vi "Post-Processing VI Bin Files - LAMPS 8 Bit.vi"() -> ()   [LabVIEW 2016]
uses:
  <vilib>/Utility/config.llb/Read Key (I32).vi
  <vilib>/Utility/config.llb/Read Key (Double).vi
  <vilib>/Utility/config.llb/NI_LVConfig.lvlib
  Classes/Processing/Processing.lvclass
panel:
  in  "B Scan Select (Text Input)":i32=400
  out "Start Trim":dbl
  out "Stop Trim":dbl
  in  "A-Scan Change":i32=627
  out "BScan":u8[][](graph)
  out "Range":dbl=4.0
  out "Bits":dbl=16.0
  out "Points Per A Scan":i32=1600
  out "A-Scans Per BScan":i32=1000
  in  "Min / Max in dB (Contrast)":cluster{dbl, dbl}(slide)={-34.05144694533762, 14.823151125401928} scale=-40.0..60.0
  in  "Create 3D Data":bool=TRUE
  in  "Max":sgl=14.823152 format="%0.2f"
  in  "Min":sgl=-34.05145 format="%0.2f"
  out "Binary File Handle":refnum<file>
  in  "Create En Face Software Event":bool=TRUE
  out "En Face":sgl[][](graph)=[[-7.930091, -7.8040323, -7.973442, -8.000936, -7.8626037, -7.893125, -7.976362, -7.866958, -7.8874545, -8.053767, -7.895429, -8.001336, -8.058077, -7.9112062, -7.757364, -7.965038, -7.9575043, -8.167074, -8.054711, -8.167959, -7.8551683, -7.915979, -7.9114604, -7.864061, -8.055119, -7.9877367, -8.029805, -7.988413, -8.037094, -7.922483, -8.156847, -7.9672847, -7.8064103, -7.9114566, -7.773133, -7.9002914, -8.085471, -7.9221673, -7.957444, -7.958286, -7.698463, -8.002342, -7.989561, -7.952671, -7.984078, -7.836235, -8.0634165, -8.028308, -8.039231, -8.056543, -7.8877096, -7.9473996, -7.865986, -7.929803, -7.9396944, -7.8729186, -7.962053, -7.976538, -7.829268, -7.759593, -7.6770754, -7.917806, -7.978408, -7.7964263, -7.9014854, -7.8359327, -8.019228, -7.9651647, -7.961875, -8.0167675, -7.915086, -7.975068, -8.046566, -7.960596, -7.990237, -8.160412, -8.09407, -7.795923, -7.8977365, -7.917423, -8.06519, -7.941408, -8.036876, -7.946509, -8.009643, -7.7677317, -8.056414, -8.105821, -8.020063, -7.946077, -7.9010644, -8.056617, -8.010448, -8.0648775, -7.9236917, -7.8220835, -7.8197546, -7.8338175, -7.908895, -7.9036684, -7.9667068, -8.103706, -7.9954534, -7.9504957, -7.829475, -7.831149, -8.244316, -8.030985, -8.157568, -7.6754923, -7.9325967, -8.037667, -7.9114547, -7.946226, -7.8830395, -7.788606, -8.123245, -7.848808, -8.020647, -7.825039, -8.136002, -7.8881106, -7.840354, -7.8498588, -7.868983, -8.012706, -8.025735, -8.1118145, -7.816016, -7.8430986, -7.9750667, -8.042043, -7.820652, -7.8192554, -7.888372, -8.02898, -7.891756, -7.86369, -7.979582, -7.7987456, -8.169637, -7.8604546, -8.097469, -7.882909, -7.745224, -7.9409885, -8.008719, -7.874554, -7.934384, -7.889922, -7.9307194, -7.976539, -7.8116565, -8.037268, -7.8819757, -7.90127, -8.004612, -7.9514766, -7.6461873, -8.051855, -8.033362, -7.820009, -8.007025, -7.9113975, -7.972308, -8.075444, -7.9308887, -8.089264, -7.8016825, -7.919436, -7.94926, -7.7312274, -8.1581135, -7.806207, -7.956523, -7.9414477, -7.9876857, -7.9657526, -7.8116117, -7.8548036, -7.9839373, -7.9158034, -7.898539, -7.780124, -7.9533, -7.8764243, -7.739191, -7.80521, -8.063391, -7.9777446, -7.7854123, -7.9521074, -7.98957, -7.888753, -7.7991505, -7.9267855, -7.9612865, -7.819488, -7.865055, -8.14359, -7.7728977, -8.085733, -7.8384624, -7.743552, -7.886237, -7.9267993, -7.9535413, -7.8223243, -7.8396297, -7.870655, -8.026216, -7.7772164, -7.80645, -8.013777, -8.012371, -7.7353735, -7.935509, -7.860224, -7.9132657, -7.845752, -7.7870827, -7.958748, -8.160488, -7.869349, -7.78722, -7.955144, -7.8493533, -7.8096776, -7.986651, -7.945869, -7.935255, -8.144389, -7.9736667, -7.752922, -7.9255905, -7.974105, -7.799902, -7.6951523, -7.799085, -7.9162817, -8.017551, -7.9524965, -7.9512806, -8.165993, -7.7668185, -8.012505, -8.16206, -8.251981, -8.013035, -7.735666, -8.077859, -8.10991, -7.949526, -7.707088, -7.949591, -7.8823195, -7.816381, -8.034339, -7.868784, -7.89056, -7.8687153, -8.057175, -7.9518924, -7.9154468, -7.939955, -7.814576, -8.049959, -7.9097743, -7.863441, -7.846818, -7.96588, -7.789853, -8.094775, -7.7202816, -8.046873, -8.085813, -7.9780364, -7.9041257, -7.926487, -7.9343805, -8.040627, -7.830686, -8.070694, -7.8358226, -7.7780213, -7.8480616, -8.064976, -8.037013, -7.7728744, -8.012946, -7.9755006, -7.906261, -8.043798, -7.911961, -7.992775, -8.001271, -7.9195423, -8.082046, -8.020159, -7.9112606, -7.775108, -8.003549, -7.9803247, -7.8879714, -8.073655, -7.8865504, -7.783486, -7.8546762, -8.020269, -8.023449, -8.067884, -7.7598515, -7.90917, -8.069023, -7.7864647, -7.870191, -7.870761, -7.9444532, -7.993182, -7.917858, -8.03805, -7.93978, -7.7982545, -7.974645, -8.004379, -7.993704, -7.819672, -8.089255, -7.9242916, -7.907874, -7.9370337, -7.863256, -7.7989616, -7.80284, -8.006147, -7.823976, -7.995604, -8.050512, -7.964656, -8.11802, -7.9949827, -7.951066, -7.7912025, -7.927686, -8.008126, -7.891107, -8.10944, -8.134752, -7.8064127, -7.910995, -8.09849, -7.8788795, -8.016058, -7.8636923, -7.9307437, -7.974993, -7.991549, -7.974662, -7.93784, -7.7311897, -8.182317, -7.7587895, -8.095182, -7.874478, -7.813459, -7.879261, -7.829288, -8.035134, -7.861396, -7.986878, -7.782207, -7.79948, -7.9310637, -7.852276, -7.9916263, -7.9213424, -8.203527, -7.921085, -8.025147, -7.8967156, -7.8208995, -7.9961405, -8.083003, -7.98257, -7.9804964, -7.8674, -8.060883, -7.9558725, -7.945471, -8.142715, -8.087639, -8.218578, -8.243896, -7.959839, -7.9356184, -7.7503934, -8.0898695, -7.868658, -7.692663, -7.887905, -7.8621182, -7.9225054, -7.836562, -8.054047, -7.982782, -7.744281, -7.963519, -8.0447, -7.849429, -7.838456, -8.119481, -7.7900977, -7.9761267, -7.8695583, -7.76462, -7.970638, -7.9605556, -7.964503, -7.9509263, -7.86703, -8.055239, -7.884155, -7.844713, -7.856759, -7.9913874, -8.0371475, -7.938692, -8.049144, -8.021844, -7.7414804, -7.920646, -8.197608, -7.880194, -7.9744005, -8.035382, -8.069501, -8.181021, -8.0188465, -8.004074, -8.031586, -8.0189085, -8.058473, -7.9364552, -7.719303, -7.905371, -7.790757, -8.214631, -7.9018154, -7.987326, -7.9526286, -7.8612223, -7.9100804, -8.08193, -7.9836636, -8.027385, -8.095275, -7.9418774, -7.9966297, -7.9296713, -8.01897, -7.9224367, -7.8740377, -7.8067255, -8.113648, -7.965984, -7.919392, -7.9538283, -7.9669385, -7.9489245, -7.9807835, -8.049196, -8.2190485, -7.967722, -8.009465, -7.814837, -7.9246864, -7.923164, -7.990351, -7.917373, -8.095252, -8.055175, -8.003493, -7.828865, -7.96325, -7.9371457, -7.87614, -7.833712, -8.081883, -7.9843564, -7.8006735, -7.917411, -7.8912277, -7.9116125, -8.126464, -7.9357214, -7.9421554, -7.757199, -7.938931, -7.852307, -8.009288, -7.8433046, -7.8127127, -7.774231, -7.958359, -7.8807616, -8.237229, -8.159578, -7.96494, -8.140689, -7.666607, -7.9215274, -7.7746763, -7.9678416, -8.0088625, -7.897964, -7.9378257, -8.099062, -8.039701, -7.9717793, -8.185365, -8.0567465, -7.9489536, -7.8975363, -8.023378, -7.8149986, -7.7747483, -8.115946, -8.063846, -7.8867245, -7.9420667, -7.8944864, -8.023156, -7.8669634, -7.876997, -7.841495, -7.9707136, -7.9111295, -7.863631, -8.016624, -7.956105, -7.858278, -8.059558, -8.096037, -7.892564, -7.9129233, -7.79077, -7.9832497, -7.985417, -7.7849727, -8.001589, -7.7398777, -7.7428336, -7.906874, -8.126725, -8.015352, -8.038417, -7.965966, -7.911179, -7.9052196, -7.9147563, -7.75231, -8.021024, -7.8436966, -8.057442, -7.9307613, -7.822249, -8.146226, -8.007187, -7.6794977, -7.83178, -7.8921013, -8.013386, -8.003119, -7.9583955, -7.938617, -8.110327, -8.210196, -7.9229064, -7.970181, -7.8199425, -8.0372505, -7.8034477, -7.8715796, -8.105112, -7.8673153, -7.9806876, -7.944533, -7.8558373, -8.031324, -8.0394125, -7.9362345, -7.8742948, -8.004431, -7.9117155, -7.92383, -8.22453, -7.9384084, -8.046981, -7.948592, -7.9943843, -8.039814, -7.867514, -7.8567586, -7.7503667, -8.132967, -7.8055544, -8.099513, -8.015846, -7.80609, -8.167438, -7.801515, -7.9792643, -7.9695144, -7.709452, -7.8683558, -7.7977037, -7.904273, -7.790883, -8.073817, -8.044217, -7.6886067, -7.854426, -7.841001, -7.8545475, -8.139268, -7.948963, -7.89186, -7.8355184, -7.917378, -7.9529567, -7.8986993, -7.7398877, -7.946703, -7.9786987, -8.031789, -7.9741163, -7.870274, -7.9702334, -8.02977, -7.8809557, -7.8097644, -7.9288607, -8.126841, -7.8123865, -7.8626604, -7.8187237, -7.8525906, -7.9653254, -7.9950914, -7.9080153, -8.03097, -7.805545, -7.777243, -7.77037, -8.001218, -8.017348, -8.007549, -7.8903728, -7.851192, -7.73721, -7.894369, -7.9804764, -7.972263, -8.017426, -7.9188137, -7.699553, -7.985173, -8.14926, -7.9460635, -7.9795494, -8.0467, -7.855538, -7.912811, -7.9511986, -7.9749317, -7.9023323, -7.9952846, -7.9592586, -8.030751, -7.920987, -7.924575, -7.641929, -7.819344, -7.847093, -7.996105, -7.60953, -7.8648734, -8.019921, -7.804081, -7.8468595, -7.806482, -7.854887, -7.9134655, -7.771183, -7.8451014, -8.077572, -8.037743, -7.8422785, -8.027252, -7.953315, -7.8755074, -7.9896126, -7.8166866, -8.076665, -7.956374, -8.030051, -7.9240355, -7.884757, -7.8483443, -7.8289475, -8.139085, -7.770633, -7.9318833, -8.016564, -7.8698854, -7.7932873, -7.8172855, -7.8905444, -7.986914, -7.9401693, -7.9614263, -7.9716263, -7.9189005, -8.085335, -7.7258472, -8.012342, -7.7290063, -7.962374, -7.736857, -7.908464, -7.95836, -7.727169, -7.9340315, -8.031877, -7.887279, -7.8412385, -8.041202, -7.8045454, -7.8905506, -7.7506995, -7.9316373, -7.9499393, -7.851978, -7.9120736, -7.9021235, -7.8550596, -7.8048263, -7.946267, -8.050364, -7.9034224, -7.9725904, -7.869547, -7.885991, -7.968221, -7.78149, -7.824945, -7.8112597, -7.997913, -8.123039, -7.8428135, -8.064973, -7.86549, -7.898531, -7.871154, -7.8630815, -8.026972, -8.056086, -8.107686, -7.9592414, -7.802565, -7.8990717, -7.8917937, -7.9946303, -7.935857, -7.7870903, -7.925476, -8.08807, -7.9506598, -7.903563, -7.7953897, -7.938492, -7.7871675, -7.921679, -7.8528447, -8.03581, -7.8427415, -7.889442, -7.972731, -8.008952, -7.9870386, -7.81934, -8.098788, -7.990713, -7.902563, -8.00334, -8.157312, -7.8009663, -7.755303, -8.165585, -8.05285, -7.908865, -7.8209777, -7.978314, -7.8780475, -7.93847, -7.8299446, -7.8623195, -7.93139, -7.7586055, -7.9444237, -7.8643084, -7.877962, -8.007582, -7.7742763, -7.890612, -8.051581, -7.892482, -7.8677154, -7.927973, -7.8819814, -7.9347353, -7.999919, -8.090686, -7.8633533, -7.88977, -8.057978, -8.034815, -7.7877083, -7.817199, -7.9679923, -8.017427, -7.9522886, -7.943636, -7.9850945, -7.99855, -7.863006, -7.88045, -8.068299, -7.925362, -8.142173, -7.8893266, -7.957223, -7.7491736, -7.852534, -8.071495, -7.865574, -7.799149, -7.8367667, -7.996641, -8.050482, -8.003815, -7.783416, -8.051039, -7.9302397, -8.008375, -7.833727, -7.8489013, -7.9530954, -7.9982214, -7.953154, -7.9360614, -8.100909, -7.979594, -7.670946, -8.022225, -7.8406134, -8.0095, -8.040179, -7.865175, -7.9610953, -8.07941, -7.9528823, -7.8656754, -7.979678, -7.802908, -7.972213, -7.9385486, -8.097144, -7.7224145, -7.8400908, -7.9734745, -8.105193, -7.8446107, -7.968687, -7.7581, -8.128169, -8.130323, -7.7925196, -8.015969, -7.678966, -7.872306, -7.836657, -7.9079814, -7.84879, -8.133352, -7.889341, -8.066047, -7.982547, -7.951533, -7.902655, -8.105811, -7.97907, -7.9479356, -7.960124, -7.8474517, -8.111724, -7.9724307, -7.975754, -7.985938, -7.9817557, -7.78798, -8.040827, -7.760837, -7.8727965, -7.984424, -8.078643, -7.885198, -7.9081254, -7.7833333, -7.908534, -7.6961055, -7.913281, -7.7185884, -8.042309, -8.115078, -8.14631, -7.806838, -7.7963495, -8.055587, -7.97538, -7.698462, -7.775273, -8.045425, -8.037591, -8.0973015, -7.7711625, -7.988266, -7.9091988, -7.8253546, -7.925254, -7.9461355, -7.766041, -7.8593016, -7.9350066, -8.008051, -7.861942, -7.8998094, -8.016808, -8.124489, -7.9874635, -8.083402, -8.1051035, -7.993055, -7.880184, -7.91285, -7.9538074, -7.9280205, -8.043174, -8.137445, -8.110672, -7.897486, -7.9666576, -7.978455, -7.9780507, -8.032585, -8.116778, -7.971109, -7.824977, -7.766515, -7.981128, -7.930899, -8.109892, -7.9214025, -7.8610687, -7.839897, -8.006488, -7.792739, -7.9065375, -8.032204, -7.81708, -7.790314, -8.064906, -8.093157, -7.839383, -8.11415, -7.9893, -8.070883, -8.176108, -7.7919936, -8.105036, -8.017701, -8.068903, -8.093538, -7.8479977, -7.9812527, -7.871276, -7.8107314, -7.958203, -7.8588, -7.829434]]
  out "error out":errorcluster
  in  "En Face Upper Depth":i32=60
  in  "En Face Lower Depth":i32=300
  in  "B-Scan Select":i32(slide) scale=0.0..1.0
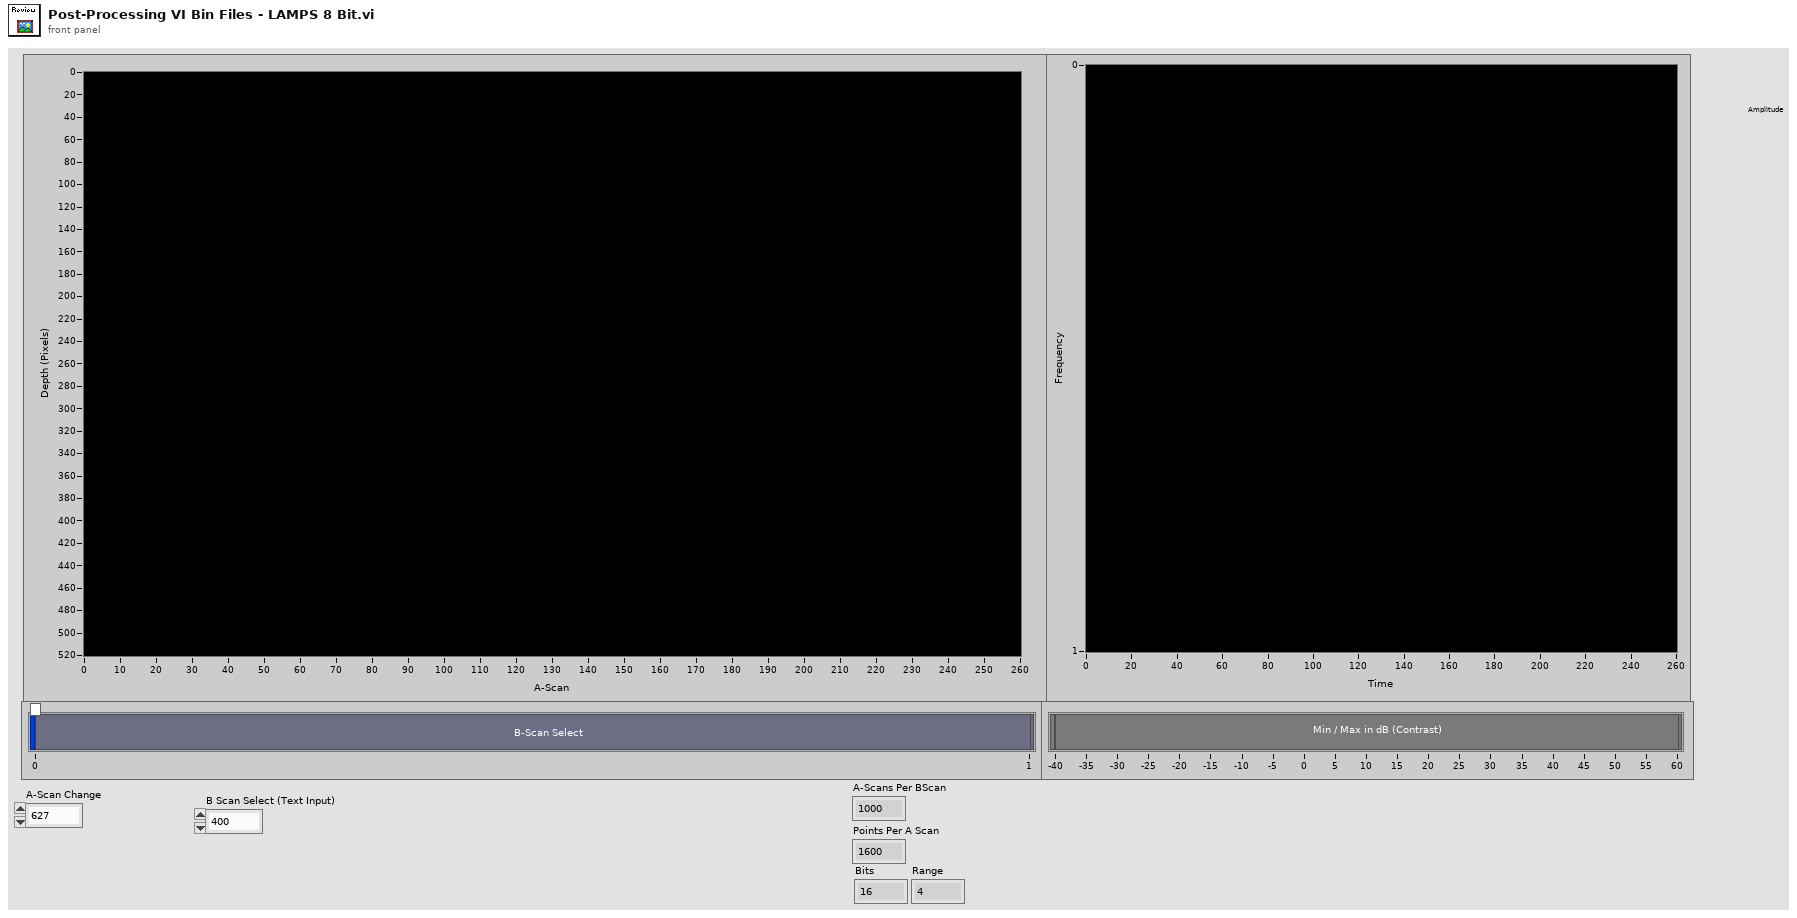
[diagram p1: front panel]
types:
  T1 = enum32{"Invalid", "Standard", "Closed", "Hidden", "Minimized", "Maximized"}
  T2 = typedef "NI_LVConfig.lvlib/Config Data RefNum.ctl" = refnum<k1>
  T3 = typedef "imagedata.ctl" = cluster{"image type":i32, "image depth":i32, "image":u8[], "mask":u8[], "colors":u32[], "Rectangle":cluster{"left":i16, "top":i16, "right":i16, "bottom":i16}}
  T4 = typedef "LVCursorListTypeDef.ctl" = cluster{"Name":string, "Color":u32, "Style":u8, "Point Style":u8, "Name Visible":bool, "Allow Drag":bool, "Cursor Mode":u32, "Plot":i32, "Index":i32, "Position":cluster{"X":dbl, "Y":dbl}, "X Scale":u32, "Y Scale":u32, "Watch Plots":i32[], "Watch All Plots":bool, "Plot Area":i32, "Label Offset":cluster{"X":dbl, "Y":dbl}}[]
  T5 = cluster{"Name":string, "Color":u32, "Style":u8, "Point Style":u8, "Name Visible":bool, "Allow Drag":bool, "Cursor Mode":u32, "Plot":i32, "Index":i32, "Position":cluster{"X":dbl, "Y":dbl}, "X Scale":u32, "Y Scale":u32, "Watch Plots":i32[], "Watch All Plots":bool, "Plot Area":i32, "Label Offset":cluster{"X":dbl, "Y":dbl}}
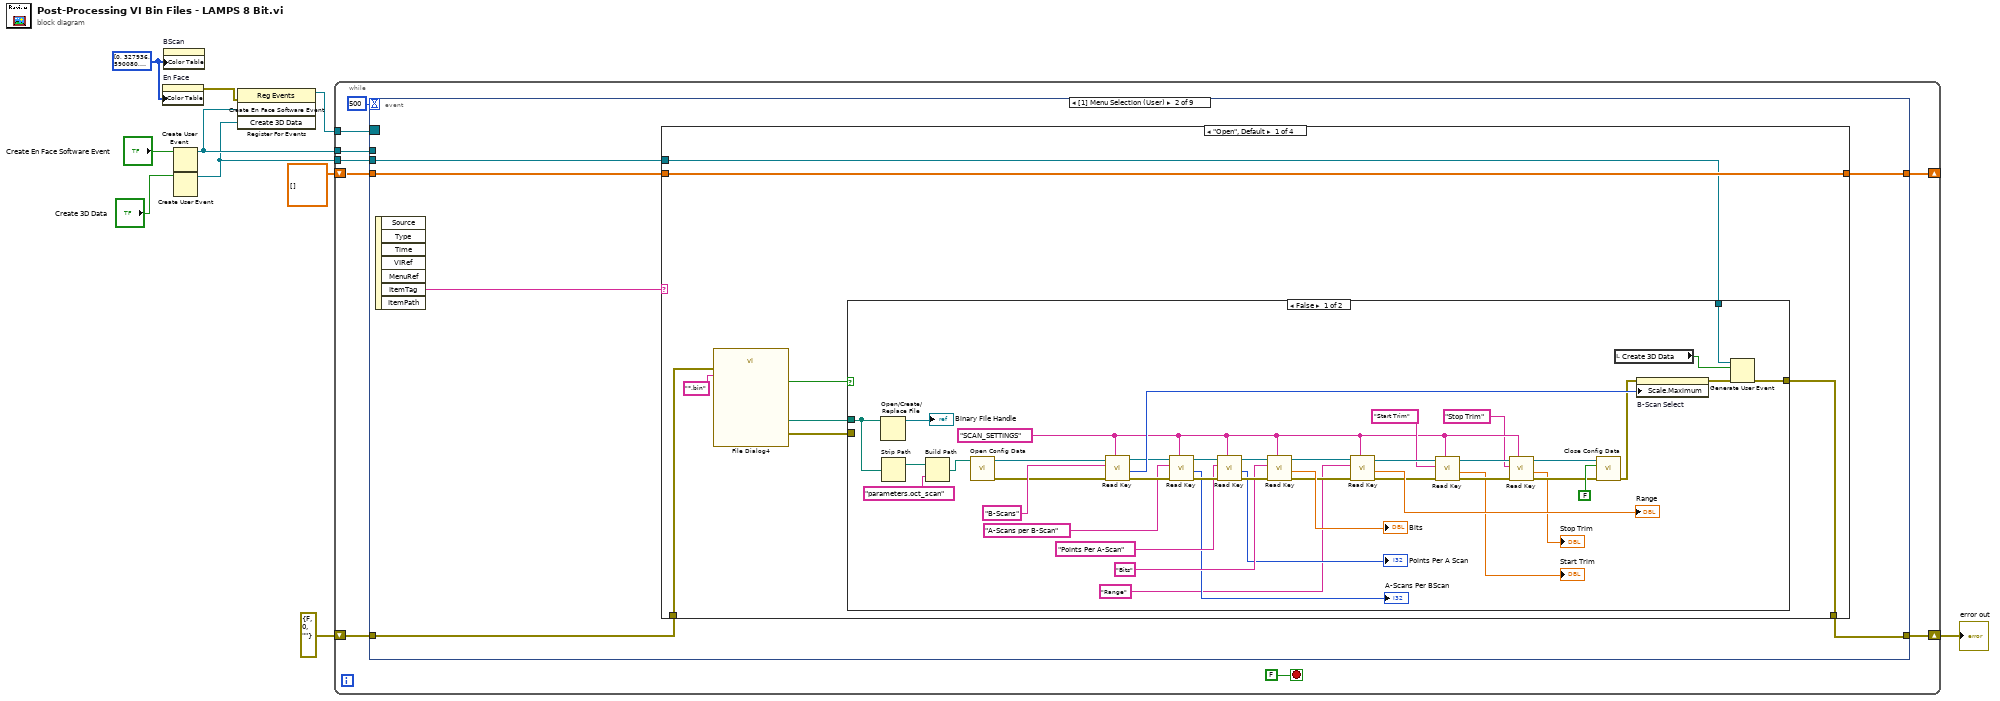
[diagram p0: block diagram]
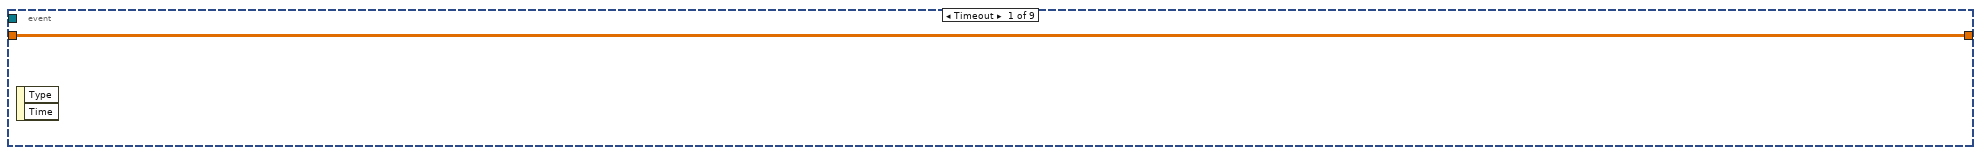
[diagram p2: hidden frame]
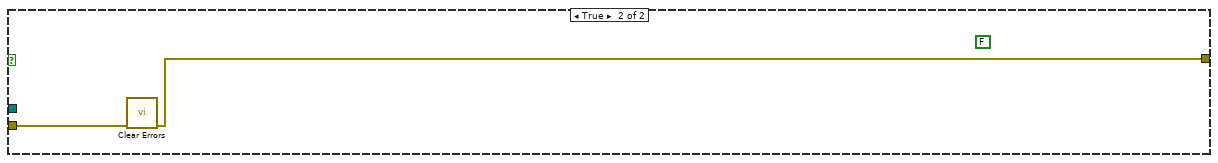
[diagram p3: hidden frame]
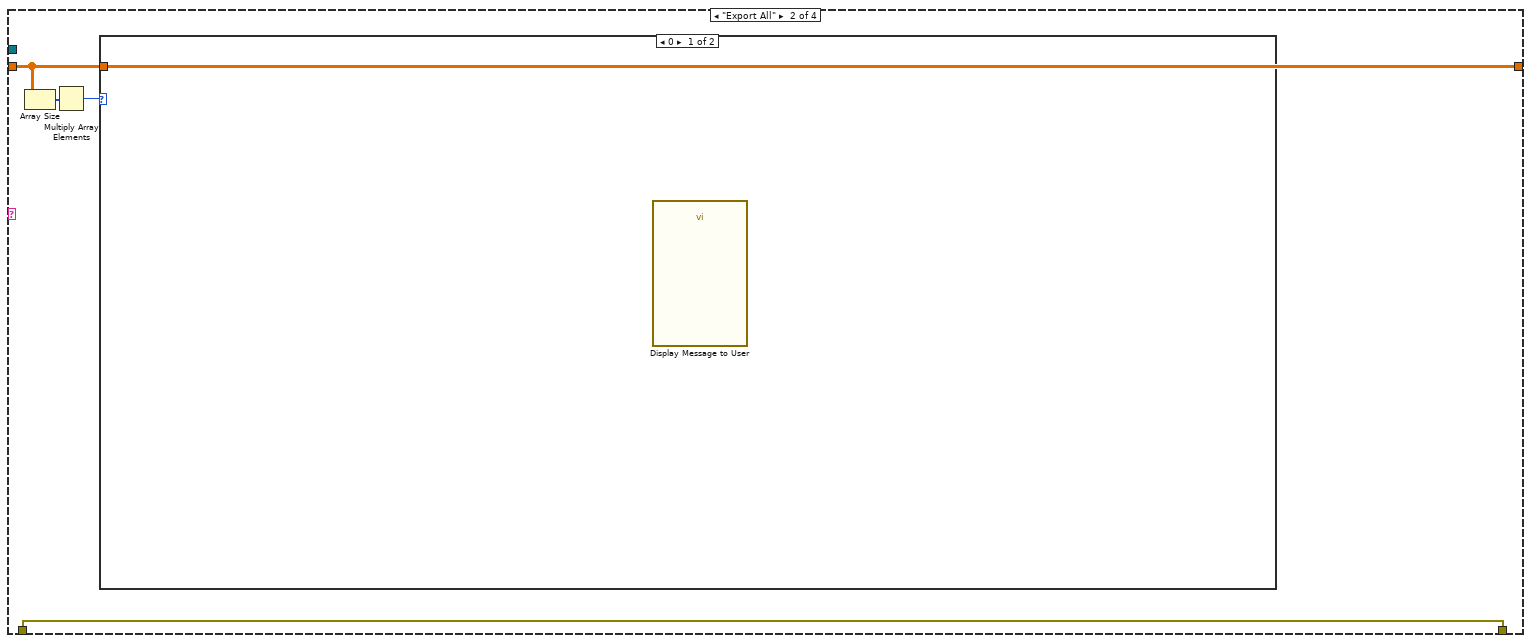
[diagram p4: hidden frame]
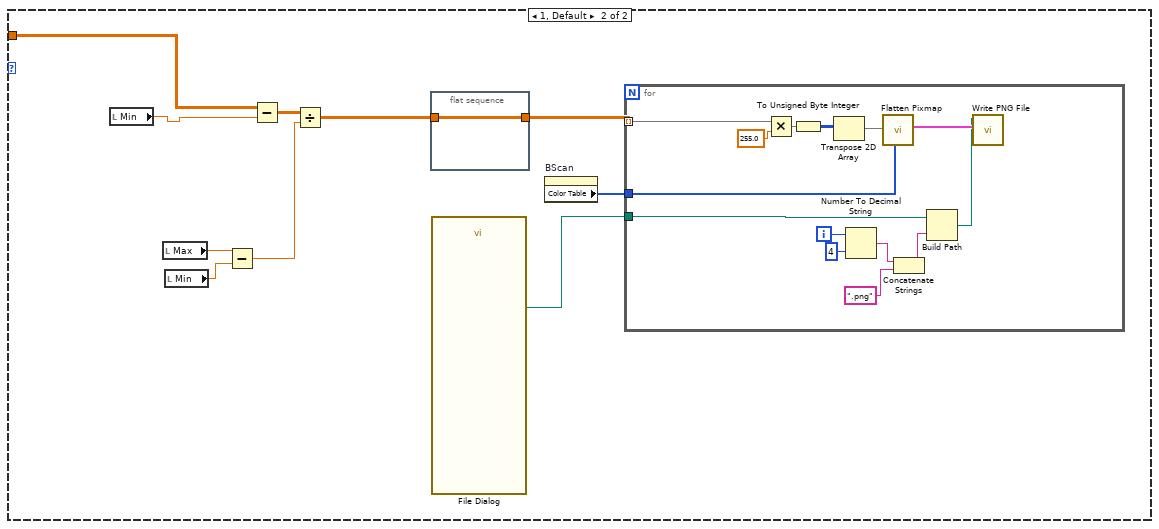
[diagram p5: hidden frame]
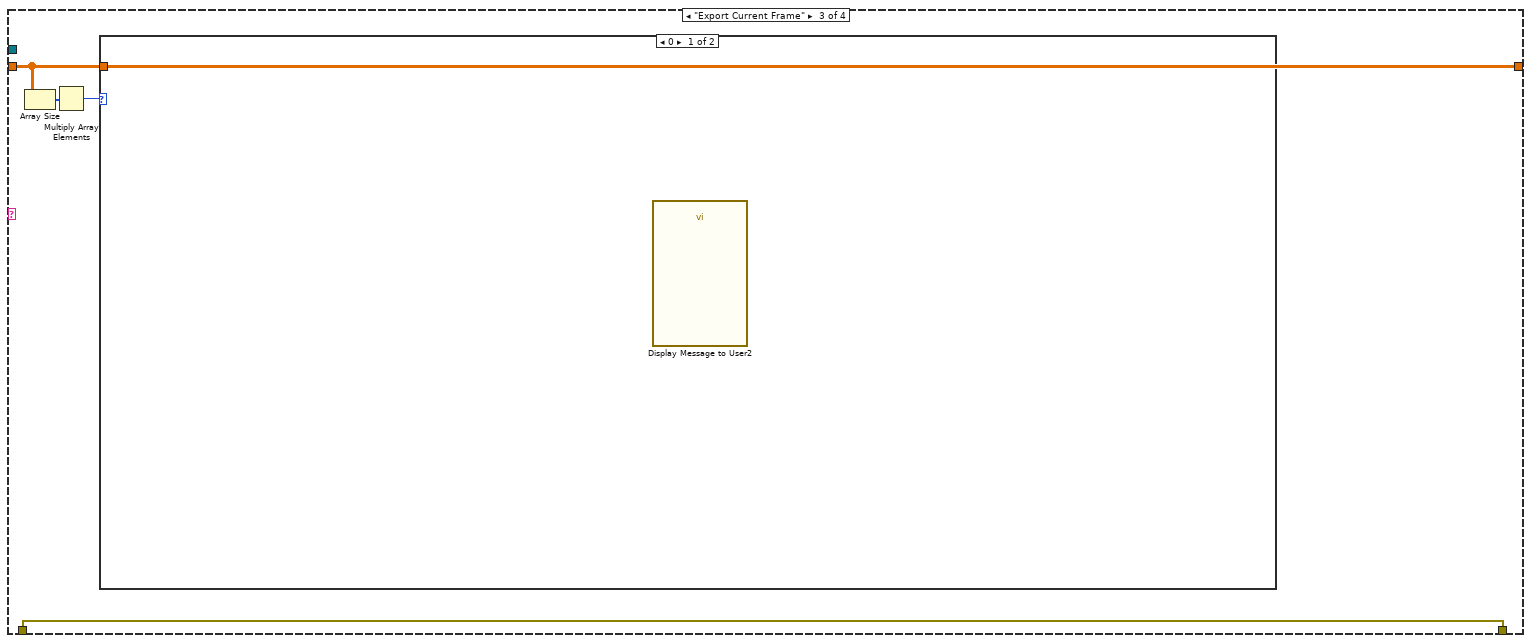
[diagram p6: hidden frame]
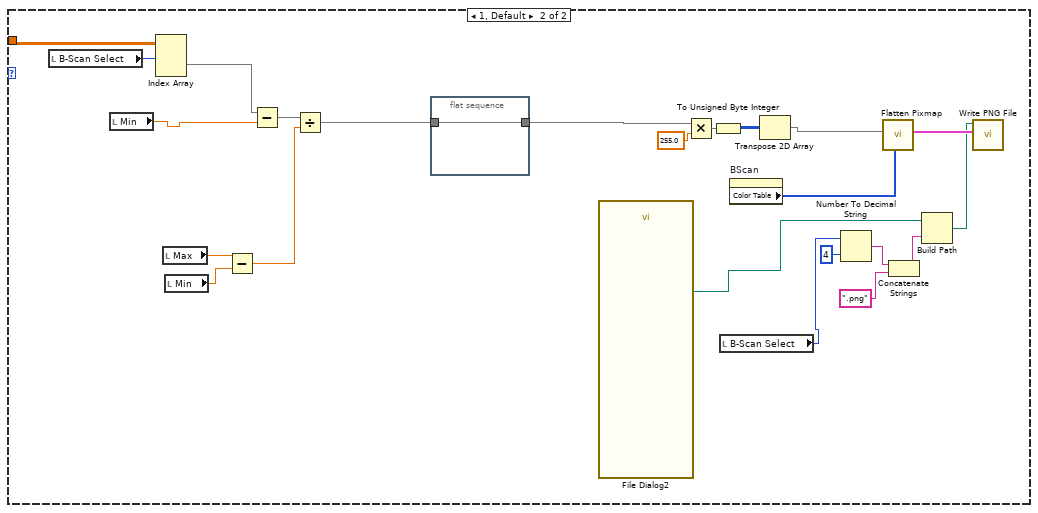
[diagram p7: hidden frame]
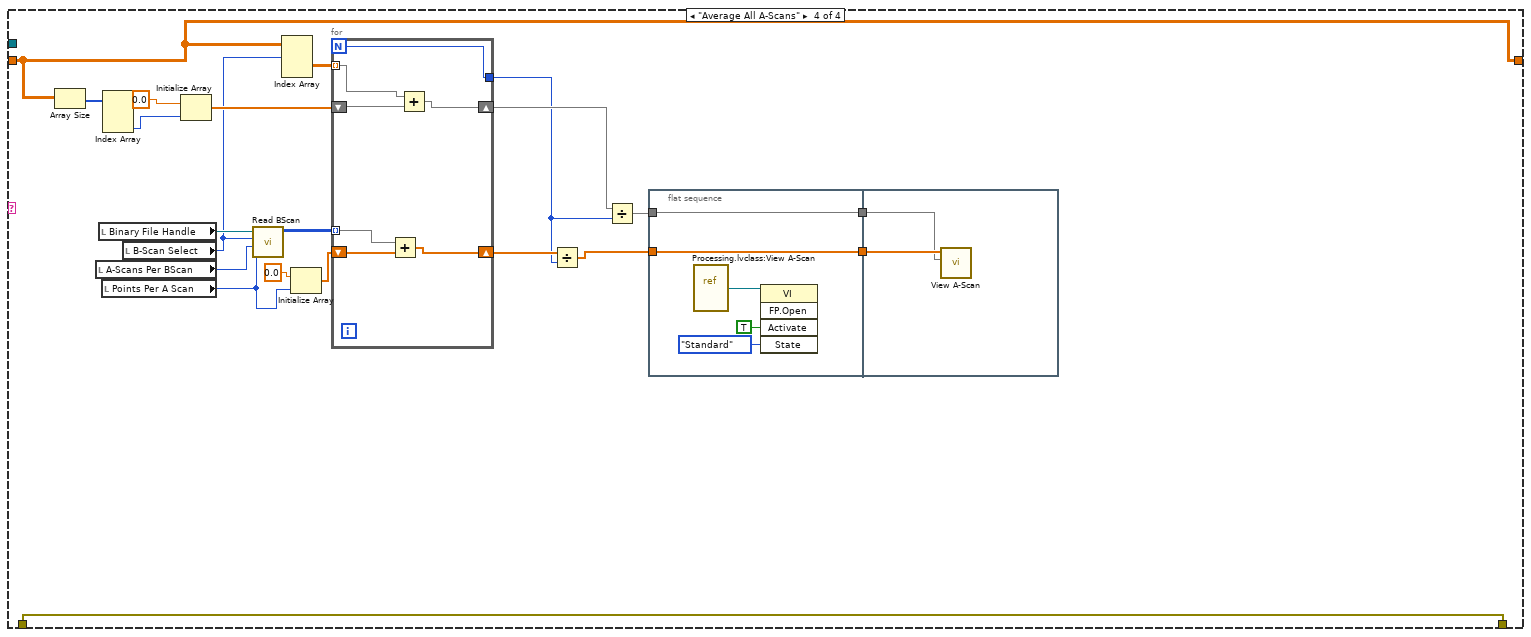
[diagram p8: hidden frame]
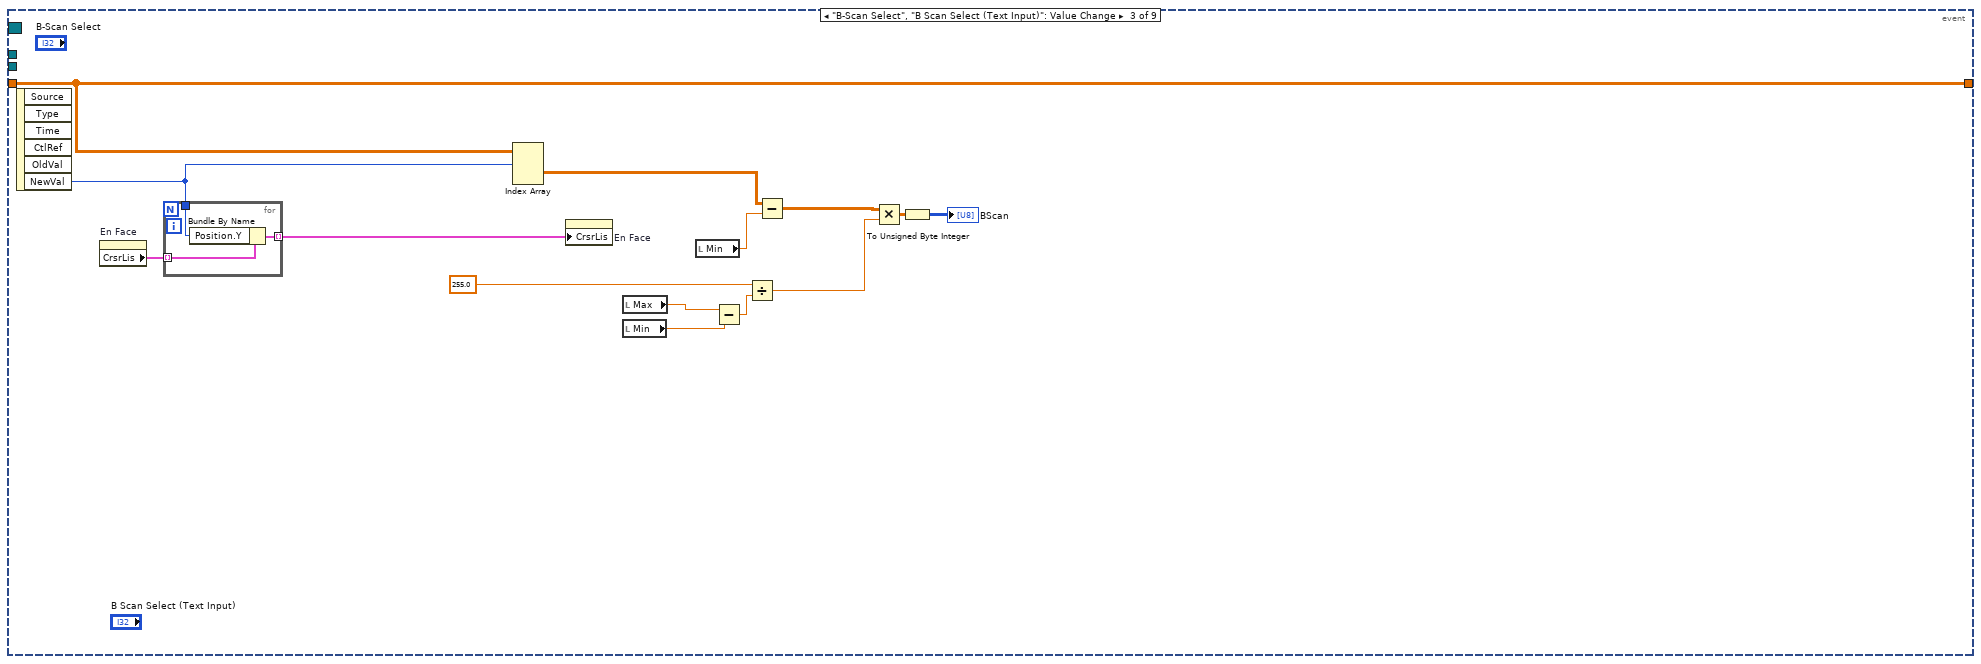
[diagram p9: hidden frame]
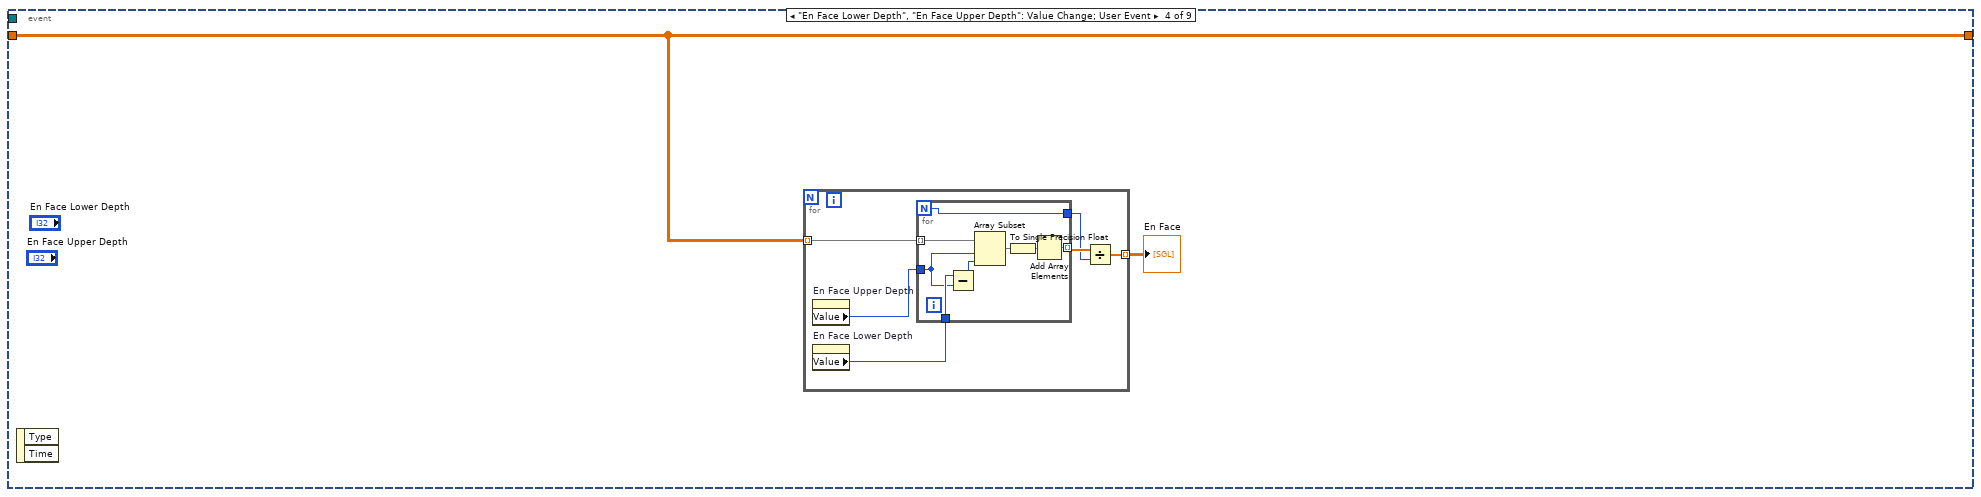
[diagram p10: hidden frame]
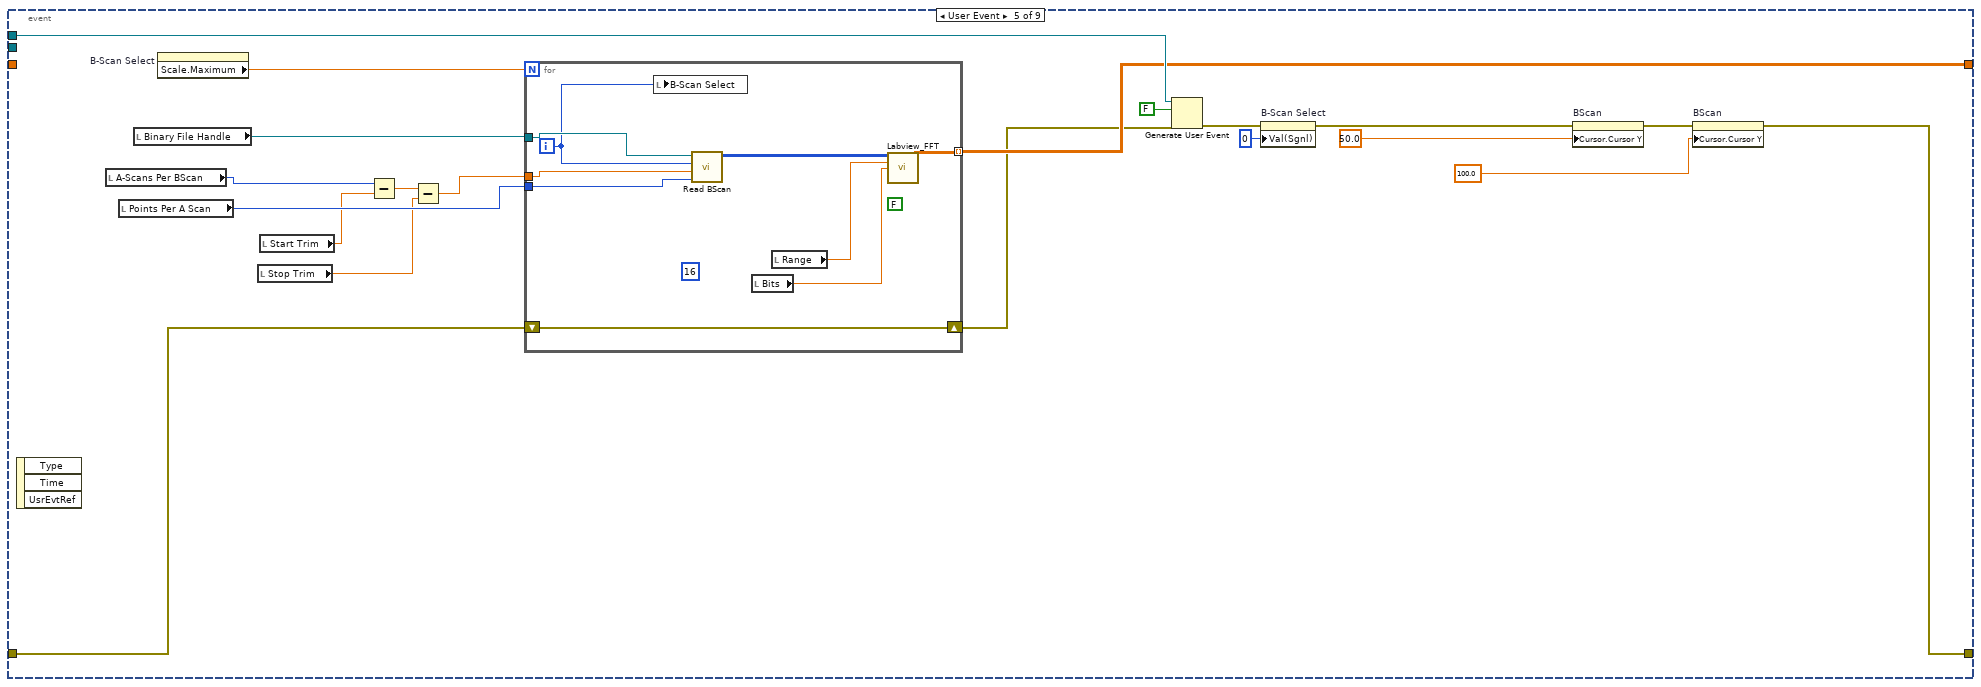
[diagram p11: hidden frame]
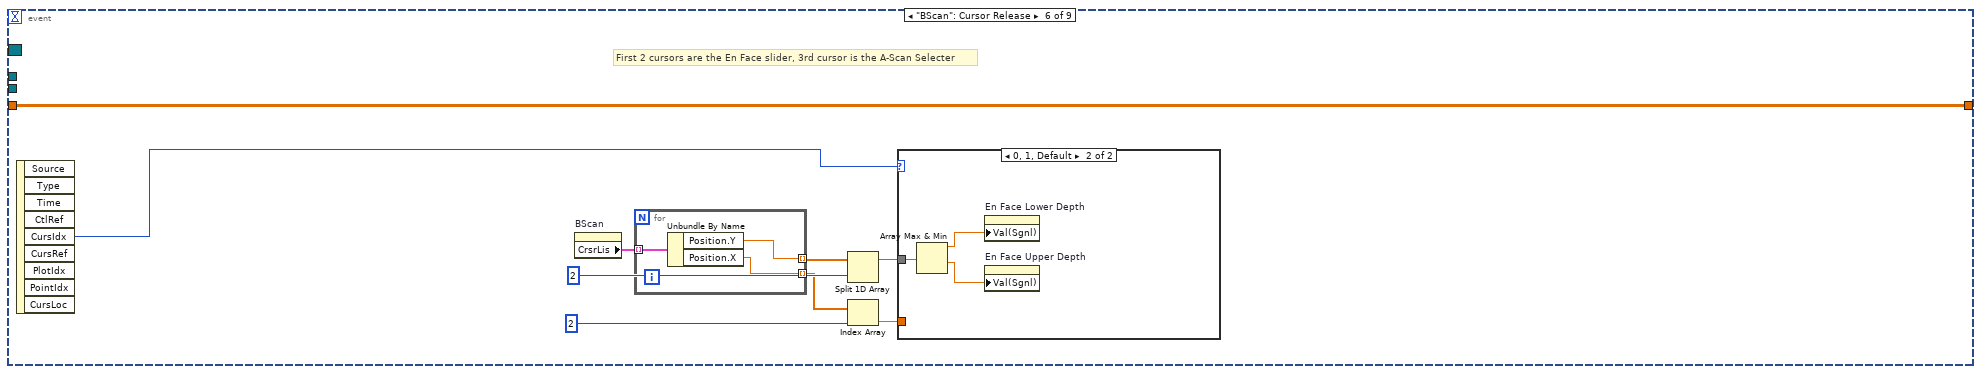
[diagram p12: hidden frame]
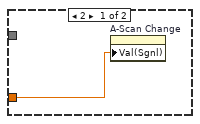
[diagram p13: hidden frame]
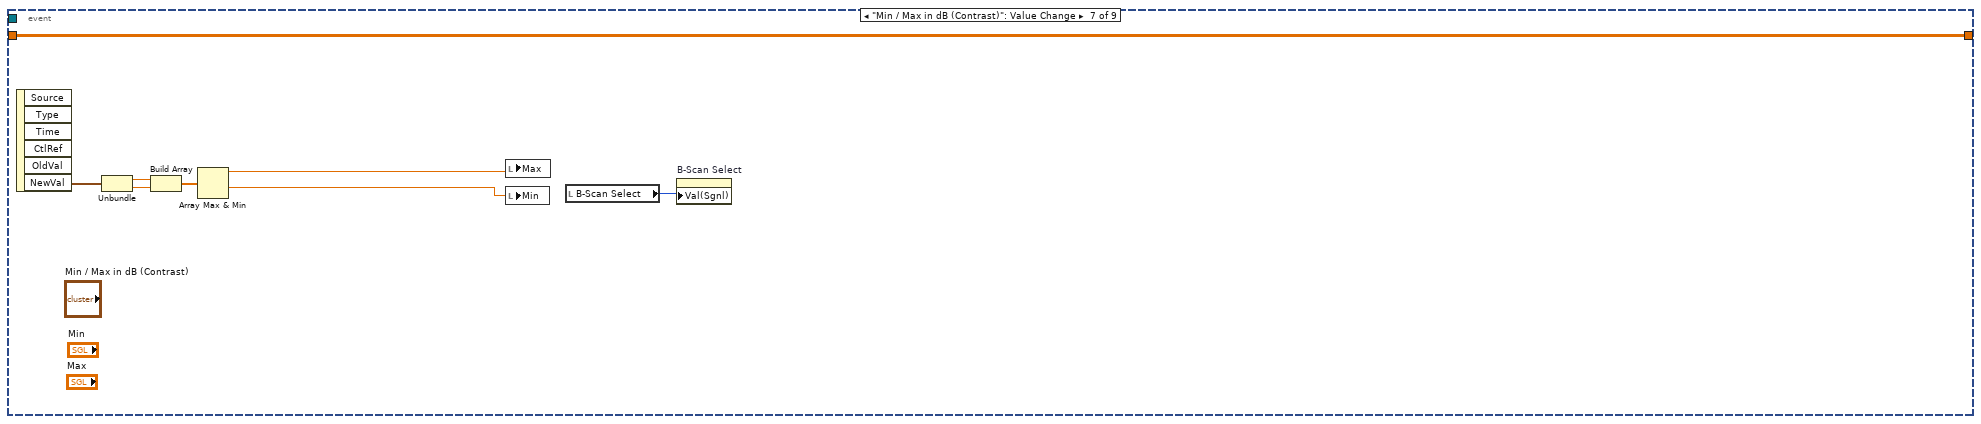
[diagram p14: hidden frame]
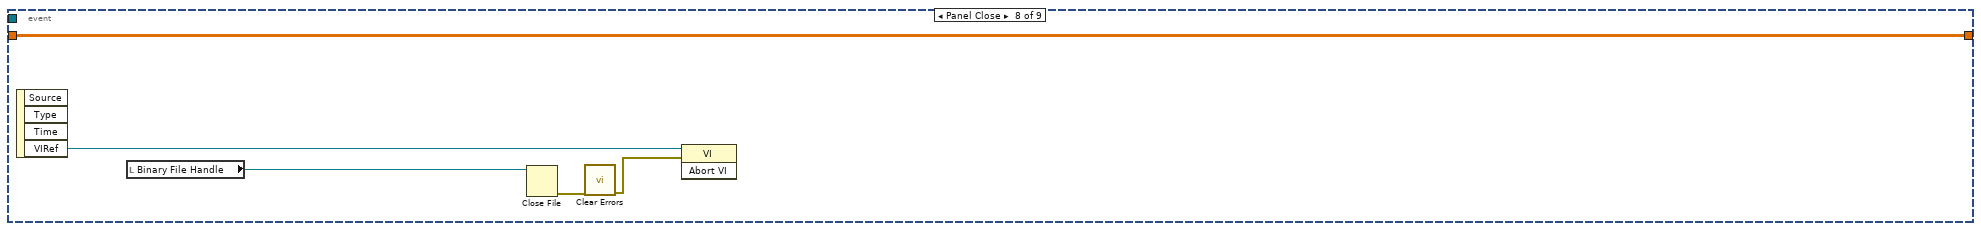
[diagram p15: hidden frame]
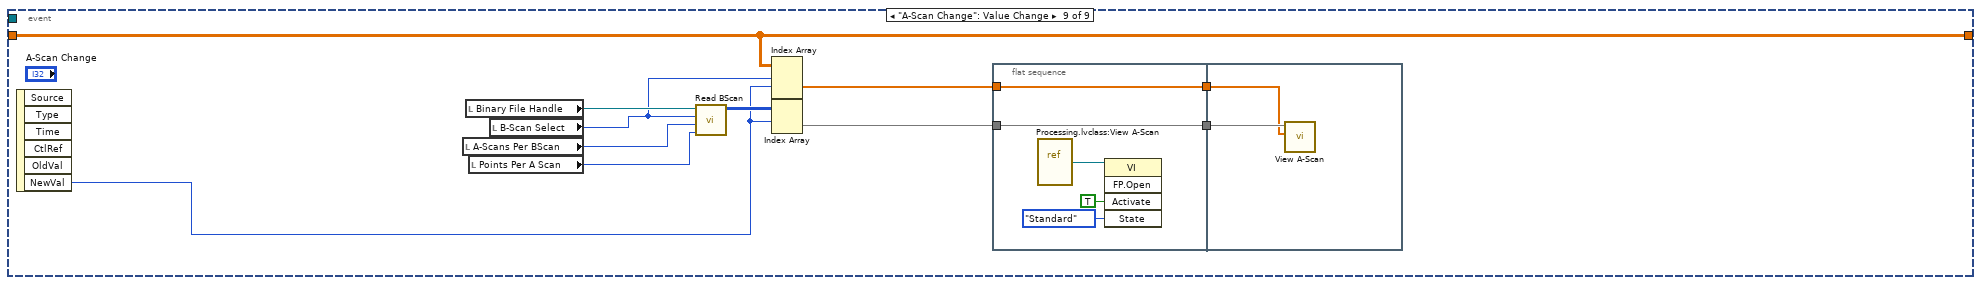
[diagram p16: hidden frame]
diagram:
  w3 = u32[] [0, 327936, 590080, 852224, 983296, 1114624, 1180160, 1311232, 1442304, 1573632, 1704704, 1770240, 1901312, 1966848, 2098176, 2163712, 2294784, 2491392, 2557184, 2688256, 2753792, 2884864, 2950656, 3081728, 3147264, 3344129, 3475457, 3540993, 3672321, 3738113, 3869185, 3934977, 4066305, 4197633, 4328961, 4394497, 4460289, 4591617, 4657409, 4788481, 4854273, 4985601, 5116929, 5248257, 5314049, 5379841, 5511169, 5576961, 5708033, 5773825, 5905153, 6036482, 6167810, 6233346, 6299138, 6430466, 6496258, 6562050, 6693634, 6759426, 6890754, 7022082, 7087874, 7153666, 7284994, 7350786, 7482114, 7547906, 7613698, 7745026, 7876354, 8007682, 8073474, 8139522, 8205314, 8336642, 8467970, 8533763, 8599555, 8665347, 8731139, 8862467, 8993795, 9059587, 9125380, 9191428, 9257220, 9388548, 9454340, 9520132, 9585924, 9717253, 9848837, 9914629, 9980165, 10045957, 10177541, 10243334, 10309126, 10375174, 10440966, 10572294, 10703623, 10769416, 10835208, 10901256, 10967049, 11033097, 11033609, 11099401, 11165450, 11231242, 11231754, 11297547, 11363339, 11429131, 11495180, 11495692, 11561740, 11693069, 11758861, 11759373, 11825165, 11891214, 11957006, 12022799, 12023311, 12089103, 12220944, 12286736, 12286736, 12352529, 12418577, 12484370, 12550162, 12615954, 12681747, 12747796, 12813588, 12813845, 12879894, 12945686, 13077015, 13142808, 13143064, 13208856, 13274905, 13340697, 13340953, 13472282, 13538075, 13604379, 13670172, 13735964, 13801757, 13867550, 13933343, 13999392, 13999648, 14065441, 14131234, 14197027, 14197541, 14263334, 14329383, 14395176, 14460969, 14592553, 14658346, 14724139, 14789932, 14790189, 14856238, 14922287, 14988080, 15053873, 15054130, 15119923, 15185972, 15251765, 15317559, 15383353, 15449146, 15449660, 15515454, 15515968, 15516226, 15582021, 15582278, 15582536, 15648587, 15648844, 15714639, 15714897, 15715155, 15780949, 15781463, 15847256, 15847770, 15848028, 15913823, 15914081, 15979875, 15980133, 15980391, 16046441, 16046444, 16046703, 16046705, 16112500, 16113015, 16113274, 16113277, 16179072, 16179330, 16179588, 16245384, 16245387, 16245389, 16245648, 16311443, 16376982, 16377241, 16377499, 16443294, 16443553, 16443555, 16443815, 16509866, 16510124, 16510127, 16575923, 16575924, 16576182, 16576441, 16576443, 16576702, 16576705, 16576963, 16577222, 16577224, 16577482, 16577485, 16577743, 16577745, 16578004, 16578262, 16578264, 16578523, 16578782, 16579040, 16579299, 16579301, 16579303, 16579562, 16579821] ("Color Table")
  n1 = property on="En Face" class="IntGraph (strict)"("Color Table"=w3) -> (error out=w2:errorcluster)  [unwired: 2 in, 1 out]
  n2 = property on="BScan" class="IntGraph (strict)"("Color Table"=w3) -> ()  [unwired: 2 in, 2 out]
  n3 = Create User Event(user event datatype="Create En Face Software Event") -> (user event=w9:refnum<user-event>)  [unwired: 1 in, 1 out]
  n4 = Create User Event(user event datatype="Create 3D Data") -> (user event=w8:refnum<user-event>)  [unwired: 1 in, 1 out]
  n5 = register-events(error in=w2, w9, w8) -> (reference out=w10:refnum<event-registration>)  [unwired: 1 in, 1 out]
  n6 = while {
    tunnel: w10 -> [w17]
    tunnel: w9 -> [w16]
    tunnel: w8 -> [w15]
    shift-right: [w13] -> w4
    shift-left: errorcluster {"status"=FALSE, "code"=0, "source"=""} ("error constant") -> [w14]
    shift-right: [w11] -> _
    shift-left: sgl[][][] [] ("Int B-Scan Channel A") -> [w12]
    stop <- FALSE stop-if-true
    n7 = event shown="[1] Menu Selection (User)" {
      selector: w17 -> [_ _ _ _ _ _ _ _ _]
      dyn-events: _ -> [_ _ _ _ _ _ _ _ _]
      timeout: 500 -> [_ _ _ _ _ _ _ _ _]
      tunnel: w15 -> [_ w23 _ _ _ _ _ _ _]
      tunnel: w16 -> [_ _ _ _ w220 _ _ _ _]
      tunnel: w14 -> [_ w22 _ _ w219 _ _ _ _]
      tunnel: [_ w21 _ _ w212 _ _ _ _] -> w13
      tunnel: w12 -> [w20 w25 w172 w188 _ w241 w249 w260 w268]
      tunnel: [w20 w24 w172 w188 w216 w241 w249 w260 w268] -> w11
      event Timeout {
        n8 = event-data() -> ()  [unwired: 1 in, 2 out]
      }
      event Menu Selection (User) {
        n9 = event-data() -> ("ItemTag"=w26:string)  [unwired: 1 in, 6 out]
        n10 = case shown="\"Open\", Default" w26 {
          tunnel: w25 -> [w34 w81 w110 w149]
          tunnel: [w34 w81 w110 w149] -> w24
          tunnel: w23 -> [w28 _ _ _]
          tunnel: w22 -> [w31 w82 w111 w156]
          tunnel: [w27 w82 w111 w156] -> w21
          frame "Open", Default {
            n11 = call "File Dialog4"("error in"=w31, "pattern (all files)"="*.bin") -> ("selected path"=w32:path, "cancelled"=w30:bool, "error out"=w29:errorcluster)  [unwired: 10 in, 1 out]
            n12 = case shown="False" w30 {
              tunnel: [w48 w77] -> w27
              tunnel: w32 -> [w75 _]
              tunnel: w29 -> [_ w78]
              tunnel: w28 -> [w47 _]
              frame False {
                w40 = "SCAN_SETTINGS" ("section")
                n13 = Open/Create/Replace File(file path (use dialog)=w75) -> (refnum out=→"Binary File Handle":refnum<file>)  [unwired: 5 in, 2 out]
                n14 = Strip Path(path=w75) -> (stripped path=w74:path)  [unwired: 1 out]
                n15 = Build Path(base path=w74, name or relative path="parameters.oct_scan") -> (appended path=w72:path)
                n16 = call <vilib>:"Open Config Data.vi"("configuration file path"=w72) -> ("error out"=w70:errorcluster, "refnum"=w69:T2)  [unwired: 8 in, 1 out]
                n17 = call-poly <vilib>:"Read Key.vi"("section"=w40, "error in (no error)"=w70, "key"="B-Scans", "refnum"=w69) -> ("error out"=w66:errorcluster, "value"=w68:i32, "refnum out"=w65:T2)  [unwired: 4 in, 1 out]
                n18 = call-poly <vilib>:"Read Key.vi"("section"=w40, "error in (no error)"=w66, "key"="A-Scans per B-Scan", "refnum"=w65) -> ("error out"=w63:errorcluster, "value"=→"A-Scans Per BScan":i32, "refnum out"=w62:T2)  [unwired: 4 in, 1 out]
                n19 = call-poly <vilib>:"Read Key.vi"("section"=w40, "error in (no error)"=w63, "key"="Points Per A-Scan", "refnum"=w62) -> ("error out"=w60:errorcluster, "value"=→"Points Per A Scan":i32, "refnum out"=w59:T2)  [unwired: 4 in, 1 out]
                n20 = call-poly <vilib>:"Read Key.vi"("section"=w40, "error in (no error)"=w60, "key"="Bits", "refnum"=w59) -> ("error out"=w52:errorcluster, "value"=→"Bits":dbl, "refnum out"=w53:T2)  [unwired: 4 in, 1 out]
                n21 = call-poly <vilib>:"Read Key.vi"("section"=w40, "error in (no error)"=w52, "key"="Range", "refnum"=w53) -> ("error out"=w45:errorcluster, "value"=→"Range":dbl, "refnum out"=w44:T2)  [unwired: 4 in, 1 out]
                n22 = call-poly <vilib>:"Read Key.vi"("section"=w40, "error in (no error)"=w45, "key"="Start Trim", "refnum"=w44) -> ("error out"=w42:errorcluster, "value"=→"Start Trim":dbl, "refnum out"=w41:T2)  [unwired: 4 in, 1 out]
                n23 = call-poly <vilib>:"Read Key.vi"("section"=w40, "error in (no error)"=w42, "key"="Stop Trim", "refnum"=w41) -> ("error out"=w38:errorcluster, "value"=→"Stop Trim":dbl, "refnum out"=w39:T2)  [unwired: 4 in, 1 out]
                n24 = call <vilib>:"Close Config Data.vi"("error in (no error)"=w38, "write file if changed (T)"=FALSE, "refnum"=w39) -> ("error out"=w57:errorcluster)  [unwired: 7 in, 1 out]
                n25 = local read "Create 3D Data"() -> (w46:bool)
                n26 = property on="B-Scan Select" class="Slide (strict)"(error in=w57, "Scale.Maximum"=w68) -> (error out=w49:errorcluster)  [unwired: 1 in, 1 out]
                n27 = Generate User Event(user event=w47, event data cluster=w46, error in=w49) -> (error out=w48:errorcluster)  [unwired: 1 in, 1 out]
              }
              frame True {
                (unwired) FALSE ("Create 3D Data")
                n28 = call <vilib>:"Clear Errors.vi"("error in (no error)"=w78) -> ("error out"=w77:errorcluster)  [unwired: 5 in, 1 out]
              }
            }
          }
          frame "Export All" {
            n29 = Array Size(array=w81) -> (size(s)=w80:i32[])
            n30 = Multiply Array Elements(1:w80) -> (0:w79:i32)
            n31 = case shown="0" w79 {
              tunnel: w81 -> [_ w92]
              frame 0 {
                n32 = call "Display Message to User"() -> ()  [unwired: 10 in, 2 out]
              }
              frame 1, Default {
                n33 = local read "Min"() -> (w86:sgl)
                n34 = local read "Max"() -> (w85:sgl)
                n35 = local read "Min"() -> (w84:sgl)
                n36 = Subtract(x=w85, y=w84) -> (x-y=w90:sgl)
                n37 = Subtract(x=w92, y=w86) -> (x-y=w91:sgl[][][])
                n38 = Divide(x=w91, y=w90) -> (x/y=w89:sgl[][][])
                n39 = flat-sequence {
                  tunnel: [w107] -> w88
                  tunnel: w89 -> [w107]
                  frame #0 {
                  }
                }
                n40 = call "File Dialog"() -> ("selected path"=w87:path)  [unwired: 12 in, 3 out]
                n41 = property on="BScan" class="IntGraph (strict)"() -> ("Color Table"=w83:u32[])  [unwired: 2 in, 2 out]
                n42 = for {
                  tunnel: w88 -> [w106] mode=indexing
                  tunnel: w87 -> [w100]
                  tunnel: w83 -> [w93]
                  i -> [w103]
                  n43 = Multiply(x=w106, y=sgl 255.0) -> (x*y=w104:sgl[][])
                  n44 = To Unsigned Byte Integer(number=w104) -> (unsigned 8bit integer=w95:u8[][])
                  n45 = Transpose 2D Array(2D array=w95) -> (transposed array=w94:u8[][])
                  n46 = Number To Decimal String(number=w103, width (-)=i16 4) -> (decimal integer string=w98:string)
                  n47 = call <vilib>:"Flatten Pixmap.vi"("colors"=w93, "8-bit pixmap"=w94) -> ("image data"=w101:T3)  [unwired: 9 in]
                  n48 = Concatenate Strings(w98, ".png" ("string")) -> (w96:string)
                  n49 = Build Path(base path=w100, name or relative path=w96) -> (appended path=w99:path)
                  n50 = call <vilib>:"Write PNG File.vi"("image data"=w101, "path to PNG file"=w99) -> ()  [unwired: 8 in, 2 out]
                }
              }
            }
          }
          frame "Export Current Frame" {
            n51 = Array Size(array=w110) -> (size(s)=w109:i32[])
            n52 = Multiply Array Elements(1:w109) -> (0:w108:i32)
            n53 = case shown="0" w108 {
              tunnel: w110 -> [_ w117]
              frame 0 {
                n54 = call "Display Message to User2"() -> ()  [unwired: 10 in, 2 out]
              }
              frame 1, Default {
                n55 = local read "B-Scan Select"() -> (w118:i32)
                n56 = local read "Min"() -> (w129:sgl)
                n57 = Index Array(array=w117, index (dim 0)=w118) -> (element=w116:sgl[][])  [unwired: 2 in]
                n58 = local read "Max"() -> (w128:sgl)
                n59 = local read "Min"() -> (w127:sgl)
                n60 = Subtract(x=w128, y=w127) -> (x-y=w133:sgl)
                n61 = Subtract(x=w116, y=w129) -> (x-y=w134:sgl[][])
                n62 = Divide(x=w134, y=w133) -> (x/y=w132:sgl[][])
                n63 = flat-sequence {
                  tunnel: [w135] -> w131
                  tunnel: w132 -> [w135]
                  frame #0 {
                  }
                }
                n64 = call "File Dialog2"() -> ("selected path"=w130:path)  [unwired: 12 in, 3 out]
                n65 = Multiply(x=w131, y=sgl 255.0) -> (x*y=w125:sgl[][])
                n66 = To Unsigned Byte Integer(number=w125) -> (unsigned 8bit integer=w113:u8[][])
                n67 = local read "B-Scan Select"() -> (w115:i32)
                n68 = property on="BScan" class="IntGraph (strict)"() -> ("Color Table"=w114:u32[])  [unwired: 2 in, 2 out]
                n69 = Transpose 2D Array(2D array=w113) -> (transposed array=w112:u8[][])
                n70 = Number To Decimal String(number=w115, width (-)=i16 4) -> (decimal integer string=w121:string)
                n71 = call <vilib>:"Flatten Pixmap.vi"("colors"=w114, "8-bit pixmap"=w112) -> ("image data"=w123:T3)  [unwired: 9 in]
                n72 = Concatenate Strings(w121, ".png" ("string")) -> (w119:string)
                n73 = Build Path(base path=w130, name or relative path=w119) -> (appended path=w122:path)
                n74 = call <vilib>:"Write PNG File.vi"("image data"=w123, "path to PNG file"=w122) -> ()  [unwired: 8 in, 2 out]
              }
            }
          }
          frame "Average All A-Scans" {
            n75 = Array Size(array=w149) -> (size(s)=w155:i32[])
            n76 = local read "A-Scans Per BScan"() -> (w151:i32)
            n77 = local read "Binary File Handle"() -> (w152:refnum<file>)
            n78 = local read "Points Per A Scan"() -> (w136:i32)
            n79 = Index Array(array=w155) -> (element #3=w147:i32)  [unwired: 3 in, 2 out]
            n80 = local read "B-Scan Select"() -> (w146:i32)
            n81 = Initialize Array(sgl 0.0 ("element"), w147) -> (w150:sgl[])
            n82 = call "Read BScan.vi"("Points Per A Scan"=w136, "A-Scans Per BScan"=w151, "B-Scan"=w146, "Byte Stream File in"=w152) -> ("Array"=w153:u16[][])  [unwired: 7 in]
            n83 = Index Array(array=w149, index (dim 0)=w146) -> (element=w148:sgl[][])  [unwired: 2 in]
            n84 = Initialize Array(sgl 0.0 ("element"), w136) -> (w138:sgl[])
            n85 = for {
              N -> [w167]
              tunnel: w148 -> [w169] mode=indexing
              shift-right: [w168] -> w140
              shift-left: w150 -> [w170]
              tunnel: [w167] -> w139
              shift-right: [w164] -> w143
              shift-left: w138 -> [w166]
              tunnel: w153 -> [w165] mode=indexing
              n86 = Add(x=w165, y=w166) -> (x+y=w164:sgl[])
              n87 = Add(x=w169, y=w170) -> (x+y=w168:sgl[])
            }
            n88 = Divide(x=w143, y=w139) -> (x/y=w142:sgl[])
            n89 = Divide(x=w140, y=w139) -> (x/y=w141:sgl[])
            n90 = flat-sequence {
              tunnel: w141 -> [w160]
              tunnel: w142 -> [w161]
              tunnel: [w161] -> w145
              tunnel: [w160] -> w144
              tunnel: w145 -> [w163]
              tunnel: w144 -> [w162]
              frame #0 {
                n91 = vi-ref "Processing.lvclass:View A-Scan.vi"() -> (w157:refnum<vi>)
                n92 = invoke class="VI" method="FP.Open"(reference=w157, "Activate"=TRUE ("Activate?"), "State"=T1."Standard") -> ()  [unwired: 2 in, 5 out]
              }
              frame #1 {
                n93 = call "View A-Scan.vi"("A-Scan Processed"=w162, "A-Scan (Raw)"=w163) -> ()  [unwired: 10 in]
              }
            }
          }
        }
      }
      event "B-Scan Select", "B Scan Select (Text Input)": Value Change {
        n94 = event-data() -> ("NewVal"=w171:i32)  [unwired: 1 in, 5 out]
        n95 = property on="En Face" class="IntGraph (strict)"() -> ("CrsrLis"=w184:T4)  [unwired: 2 in, 2 out]
        n96 = for {
          tunnel: w184 -> [w187] mode=indexing
          tunnel: w171 -> [w186]
          tunnel: [w185] -> w183 mode=indexing
          n97 = Bundle By Name(cluster=w187, "Position.Y"=w186) -> (w185:T5)
        }
        n98 = Index Array(array=w172, index (dim 0)=w171) -> (element=w173:sgl[][])  [unwired: 2 in]
        n99 = property on="En Face" class="IntGraph (strict)"("CrsrLis"=w183) -> ()  [unwired: 2 in, 2 out]
        n100 = local read "Max"() -> (w181:sgl)
        n101 = local read "Min"() -> (w180:sgl)
        n102 = local read "Min"() -> (w175:sgl)
        n103 = Subtract(x=w181, y=w180) -> (x-y=w179:sgl)
        n104 = Divide(x=sgl 255.0, y=w179) -> (x/y=w177:sgl)
        n105 = Subtract(x=w173, y=w175) -> (x-y=w178:sgl[][])
        n106 = Multiply(x=w178, y=w177) -> (x*y=w176:sgl[][])
        n107 = To Unsigned Byte Integer(number=w176) -> (unsigned 8bit integer=→"BScan":u8[][])
      }
      event "En Face Lower Depth", "En Face Upper Depth": Value Change; User Event {
        n108 = event-data() -> ()  [unwired: 1 in, 2 out]
        n109 = for {
          tunnel: [w190] -> w189 mode=indexing
          tunnel: w188 -> [w191] mode=indexing
          n110 = property on="En Face Upper Depth" class="DigNum (strict)"() -> ("Value"=w195:i32)  [unwired: 2 in, 2 out]
          n111 = property on="En Face Lower Depth" class="DigNum (strict)"() -> ("Value"=w194:i32)  [unwired: 2 in, 2 out]
          n112 = for {
            N -> [w200]
            tunnel: w191 -> [w203] mode=indexing
            tunnel: w195 -> [w196]
            tunnel: w194 -> [w197]
            tunnel: [w201] -> w193 mode=indexing
            tunnel: [w200] -> w192
            n113 = Subtract(x=w197, y=w196) -> (x-y=w198:i32)
            n114 = Array Subset(array=w203, index=w196, length=w198) -> (w202:sgl[])
            n115 = To Single Precision Float(number=w202) -> (single precision float=w199:sgl[])
            n116 = Add Array Elements(numeric array=w199) -> (sum=w201:sgl)
          }
          n117 = Divide(x=w193, y=w192) -> (x/y=w190:sgl[])
        }
        "En Face" <- w189
      }
      event User Event {
        n118 = event-data() -> ()  [unwired: 1 in, 3 out]
        n119 = local read "A-Scans Per BScan"() -> (w208:i32)
        n120 = local read "Points Per A Scan"() -> (w215:i32)
        n121 = local read "Binary File Handle"() -> (w222:refnum<file>)
        n122 = property on="B-Scan Select" class="Slide (strict)"() -> ("Scale.Maximum"=w221:dbl)  [unwired: 2 in, 2 out]
        n123 = local read "Stop Trim"() -> (w205:dbl)
        n124 = local read "Start Trim"() -> (w207:dbl)
        n125 = Subtract(x=w208, y=w207) -> (x-y=w206:dbl)
        n126 = Subtract(x=w206, y=w205) -> (x-y=w204:dbl)
        n127 = for {
          N: w221 -> [_]
          tunnel: w222 -> [w232]
          tunnel: [w229] -> w216 mode=indexing
          tunnel: w204 -> [w228]
          tunnel: w215 -> [w225]
          shift-right: [w230] -> w209
          shift-left: w219 -> [w230]
          i -> [w231]
          (unwired) FALSE ("Linear?")
          (unwired) u16 16 ("Card Resolution (bits)")
          n128 = local write "B-Scan Select"(w231) -> ()
          n129 = call "Read BScan.vi"("Points Per A Scan"=w225, "A-Scans Per BScan"=w228, "B-Scan"=w231, "Byte Stream File in"=w232) -> ("Array"=w224:u16[][])  [unwired: 7 in]
          n130 = local read "Bits"() -> (w227:dbl)
          n131 = local read "Range"() -> (w226:dbl)
          n132 = call "Labview_FFT.vi"("Channel A"=w224, "Range"=w226, "Bits"=w227) -> ("Int B-Scan Channel A"=w229:sgl[][])  [unwired: 12 in]
        }
        n133 = Generate User Event(user event=w220, event data cluster=FALSE ("event data"), error in=w209) -> (error out=w218:errorcluster)  [unwired: 1 in, 1 out]
        n134 = property on="B-Scan Select" class="Slide (strict)"(error in=w218, "Val(Sgnl)"=0 ("Value (Signaling)")) -> (error out=w214:errorcluster)  [unwired: 1 in, 1 out]
        n135 = property on="BScan" class="IntGraph (strict)"(error in=w214, "Cursor.Cursor Y"=50.0 ("Cursor.Cursor Position:Cursor Y")) -> (error out=w213:errorcluster)  [unwired: 1 in, 1 out]
        n136 = property on="BScan" class="IntGraph (strict)"(error in=w213, "Cursor.Cursor Y"=100.0 ("Cursor.Cursor Position:Cursor Y")) -> (error out=w212:errorcluster)  [unwired: 1 in, 1 out]
      }
      event "BScan": Cursor Release {
        # "First 2 cursors are the En Face slider, 3rd cursor is the A-Scan Selecter"
        n137 = event-data() -> ("CursIdx"=w237:i32)  [unwired: 1 in, 8 out]
        n138 = property on="BScan" class="IntGraph (strict)"() -> ("CrsrLis"=w240:T4)  [unwired: 2 in, 2 out]
        n139 = for {
          tunnel: w240 -> [w248] mode=indexing
          tunnel: [w247] -> w236 mode=indexing
          tunnel: [w246] -> w234 mode=indexing
          n140 = Unbundle By Name(w248) -> ("Position.Y"=w247:dbl, "Position.X"=w246:dbl)
        }
        n141 = Split 1D Array(array=w236, index=2) -> (first subarray=w238:dbl[])  [unwired: 1 out]
        n142 = Index Array(array=w234, index=2) -> (element=w233:dbl)
        n143 = case shown="0, 1, Default" w237 {
          tunnel: w238 -> [_ w243]
          tunnel: w233 -> [w242 _]
          frame 2 {
            n144 = property on="A-Scan Change" class="DigNum (strict)"("Val(Sgnl)"=w242) -> ()  [unwired: 2 in, 2 out]
          }
          frame 0, 1, Default {
            n145 = Array Max & Min(array=w243) -> (max value=w244:dbl, min value=w245:dbl)  [unwired: 2 out]
            n146 = property on="En Face Lower Depth" class="DigNum (strict)"("Val(Sgnl)"=w244) -> ()  [unwired: 2 in, 2 out]
            n147 = property on="En Face Upper Depth" class="DigNum (strict)"("Val(Sgnl)"=w245) -> ()  [unwired: 2 in, 2 out]
          }
        }
      }
      event "Min / Max in dB (Contrast)": Value Change {
        n148 = event-data() -> ("NewVal"=w256:cluster{dbl, dbl})  [unwired: 1 in, 5 out]
        n149 = Unbundle(w256) -> (w254:dbl, w255:dbl)
        n150 = Build Array(w254, w255) -> (w253:dbl[])
        n151 = Array Max & Min(array=w253) -> (max value=w251:dbl, min value=w252:dbl)  [unwired: 2 out]
        n152 = local write "Max"(w251) -> ()
        n153 = local write "Min"(w252) -> ()
        n154 = local read "B-Scan Select"() -> (w250:i32)
        n155 = property on="B-Scan Select" class="Slide (strict)"("Val(Sgnl)"=w250) -> ()  [unwired: 2 in, 2 out]
      }
      event Panel Close {
        n156 = event-data() -> ("VIRef"=w261:refnum<vi>)  [unwired: 1 in, 3 out]
        n157 = local read "Binary File Handle"() -> (w259:refnum<file>)
        n158 = Close File(refnum=w259) -> (error out=w258:errorcluster)  [unwired: 1 in, 1 out]
        n159 = call <vilib>:"Clear Errors.vi"("error in (no error)"=w258) -> ("error out"=w257:errorcluster)  [unwired: 5 in, 1 out]
        n160 = invoke class="VI" method="Abort VI"(reference=w261, error in=w257) -> ()  [unwired: 1 in, 3 out]
      }
      event "A-Scan Change": Value Change {
        n161 = event-data() -> ("NewVal"=w266:i32)  [unwired: 1 in, 5 out]
        n162 = local read "A-Scans Per BScan"() -> (w271:i32)
        n163 = local read "Binary File Handle"() -> (w272:refnum<file>)
        n164 = local read "Points Per A Scan"() -> (w270:i32)
        n165 = local read "B-Scan Select"() -> (w267:i32)
        n166 = call "Read BScan.vi"("Points Per A Scan"=w270, "A-Scans Per BScan"=w271, "B-Scan"=w267, "Byte Stream File in"=w272) -> ("Array"=w269:u16[][])  [unwired: 7 in]
        n167 = Index Array(array=w268, index (dim 0)=w267, index (dim 1)=w266) -> (element=w264:sgl[])  [unwired: 1 in]
        n168 = Index Array(array=w269, index (row)=w266) -> (element=w265:u16[])  [unwired: 1 in]
        n169 = flat-sequence {
          tunnel: w264 -> [w276]
          tunnel: w265 -> [w277]
          tunnel: [w277] -> w263
          tunnel: [w276] -> w262
          tunnel: w263 -> [w279]
          tunnel: w262 -> [w278]
          frame #0 {
            n170 = vi-ref "Processing.lvclass:View A-Scan.vi"() -> (w273:refnum<vi>)
            n171 = invoke class="VI" method="FP.Open"(reference=w273, "Activate"=TRUE ("Activate?"), "State"=T1."Standard") -> ()  [unwired: 2 in, 5 out]
          }
          frame #1 {
            n172 = call "View A-Scan.vi"("A-Scan Processed"=w278, "A-Scan (Raw)"=w279) -> ()  [unwired: 10 in]
          }
        }
      }
    }
  }
  "error out" <- w4
